vi "GRNF_Compressor.vi"(7 "RefNum Name":string="My Motor RefNum") -> (0 "Error":errorcluster, 3 "Device Reference":T1)   [LabVIEW 2019]
doc: "This VI loads compressor refnum on code boot and then stores it in memory so that the information does not have to be queried on subsequent loop cycles. This VI is configured for polymorphic use."
uses:
  <vilib>/Rock Robotics/WPI/Compressor/WPI_CompressorDevRef.ctl
  <vilib>/Rock Robotics/WPI/Utilities/WPI_GetSetVariantRefNum.vi
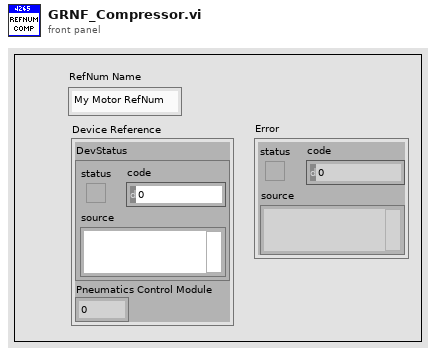
[diagram p1: front panel]
types:
  T1 = typedef "WPI_CompressorDevRef.ctl" = cluster{"DevStatus":errorcluster, "Pneumatics Control Module":u8}
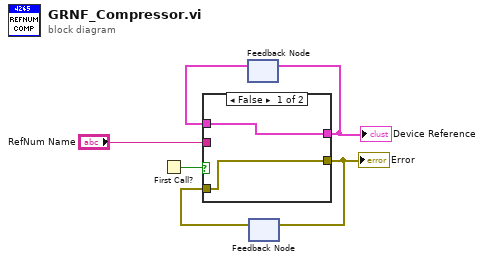
[diagram p0: block diagram]
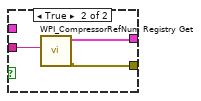
[diagram p2: hidden frame]
diagram:
  n1 = First Call?() -> (First Call?: T/F=w6:bool)
  n2 = feedback #1() -> (w5:T1)  [unwired: 1 in]
  n3 = feedback #2() -> (w1:errorcluster)  [unwired: 1 in]
  n4 = case shown="False" w6 {
    tunnel: [w8 w11] -> w4
    tunnel: w5 -> [w8 _]
    tunnel: "RefNum Name" -> [_ w10]
    tunnel: [w7 w9] -> w2
    tunnel: w1 -> [w7 _]
    frame False {
    }
    frame True {
      n5 = call <vilib>:"WPI_CompressorRefNum Registry Get.vi"("refnum name"=w10) -> ("error out"=w9:errorcluster, "CompressorDevRef"=w11:T1)  [unwired: 9 in]
    }
  }
  "Device Reference" <- w4
  "Error" <- w2
  n6 = feedback-in #1(w4) -> ()
  n7 = feedback-in #2(w2) -> ()
